vi "WSVCAP SHL Host LL Manage FPGA Top Level Controls Core.vi"(0 "Value In":variant, 1 "FPGA VI Reference (Init Only)":T2, 7 "FPGA Top Level Control":T3=enum."Read Status Flag", 11 "error in (no error)":errorcluster, 12 "Simulate FPGA (Init Only)":bool=TRUE, 13 "Operation":T4, 14 "FPGA":T1) -> (4 "Value Out":variant, 15 "error out":errorcluster)   [LabVIEW 2017]
uses:
  Type Defs/WSVCAP SHL Top Level Control Operation Enum.ctl
  Type Defs/WSVCAP SHL Top Level Control Enum.ctl
  Type Defs/WSVCAP SHL FPGA Ref.ctl
  Type Defs/WSVCAP SHL FPGA Enum.ctl
  user.lib/Utilities/Type Defs/MISC IO Choice Enum.ctl
  Type Defs/Top Level Controls Core Cluster.ctl
  Type Defs/WSVCAP SHL Gatekeeper Operation Enum.ctl
  Type Defs/WSVCAP SHL State.ctl
  Type Defs/WSVCAP SHL Transaction Enum.ctl
  <vilib>/Utility/error.llb/Error Cluster From Error Code.vi
  <vilib>/rvi/errors/niLvFpgaAdjustHostInterfaceError.vi
  <vilib>/rvi/interface/nirviReadWriteControl/nirviReadWriteControl.xnode
  FPGA Bitfiles/WSVCAPShell_WiSpryFPGA1_WSVCAPSHLFPGATLT_ffr+nD2N+rA.lvbitx
  NiFpgaLv.dll
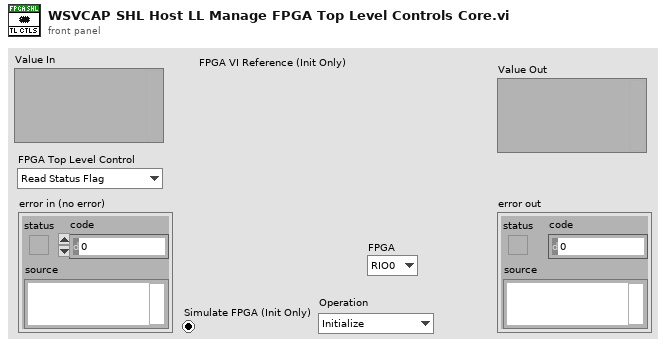
[diagram p1: front panel]
types:
  T1 = typedef "WSVCAP SHL FPGA Enum.ctl" = enum16{"RIO0", "RIO1"}
  T2 = typedef "WSVCAP SHL FPGA Ref.ctl" = refnum<k20>
  T3 = typedef "WSVCAP SHL Top Level Control Enum.ctl" = enum16{"Start", "Cmd", "Transaction", "Wait Ticks", "Socket Mask", "UUT Set", "Slave Address", "Sub Address", "Bytes to Write", "Bytes to Read", "Write Data", "Write Flag", "Read Data", "Read Flag", "Ack Read", "Read Status Flag", "Ack Read Status", "Status", "Cycle Count", "Stop Cycle", "Exit"}
  T4 = typedef "WSVCAP SHL Top Level Control Operation Enum.ctl" = enum16{"Initialize", "Set Control", "Read Control", "Close"}
  T5 = typedef "WSVCAP SHL Gatekeeper Operation Enum.ctl" = enum16{"Initialize", "Lock", "Unlock", "Close"}
  T6 = typedef "Top Level Controls Core Cluster.ctl" = cluster{"Ctl Refs":refnum<vi>[], "FPGA VI Ref":T2, "Simulate":bool}
  T7 = typedef "MISC IO Choice Enum.ctl" = enum16{"Read", "Write"}
  T8 = typedef "WSVCAP SHL State.ctl" = enum8{"Idle", "Transfer Data"}
  T9 = typedef "WSVCAP SHL Transaction Enum.ctl" = enum16{"I2C-Read Data", "I2C-Write Data", "RFFE-Ext Write", "RFFE-Ext Read"}
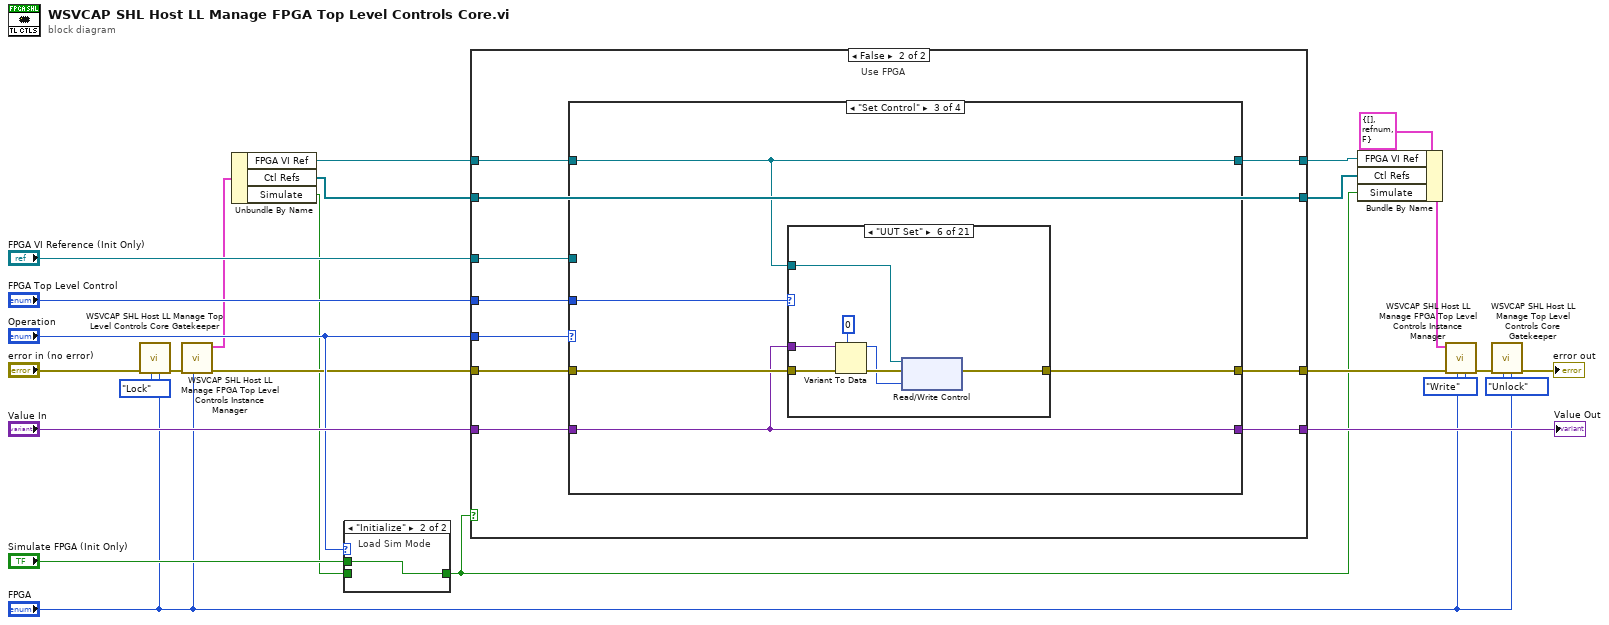
[diagram p0: block diagram]
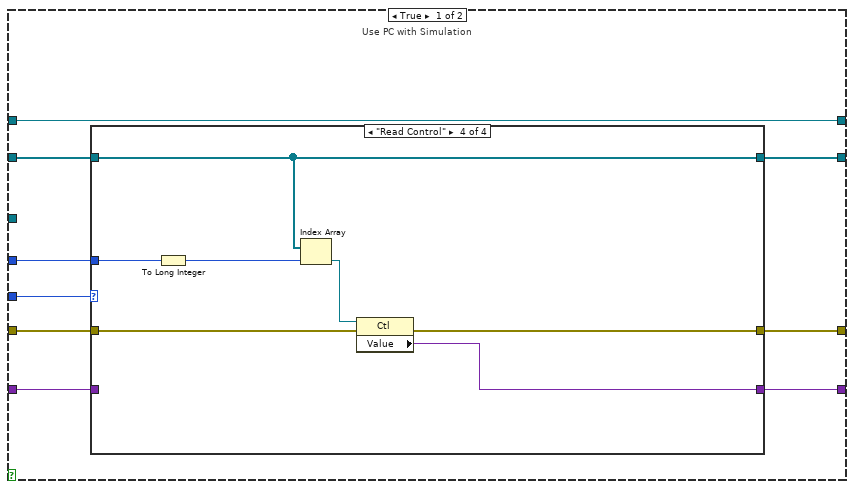
[diagram p2: hidden frame]
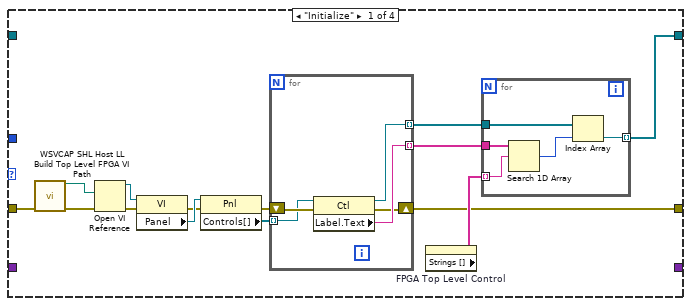
[diagram p3: hidden frame]
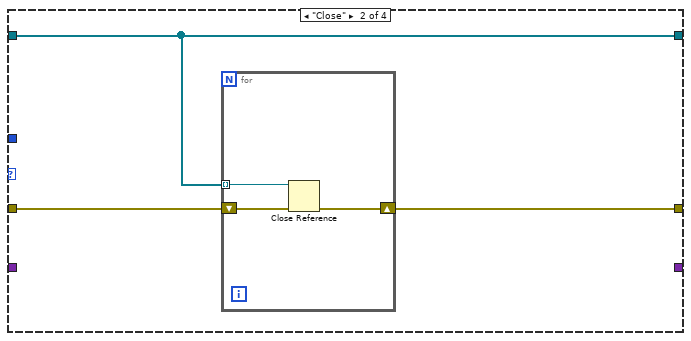
[diagram p4: hidden frame]
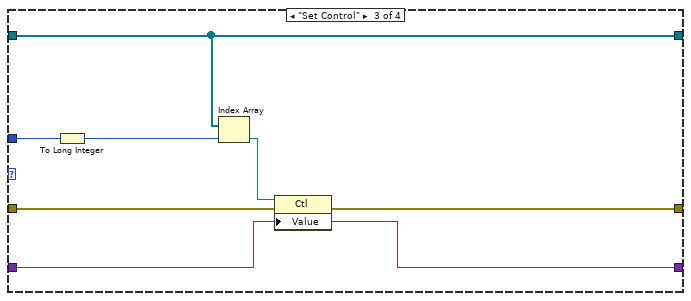
[diagram p5: hidden frame]
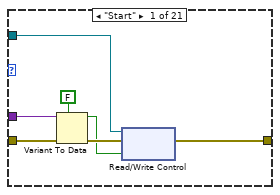
[diagram p8: hidden frame]
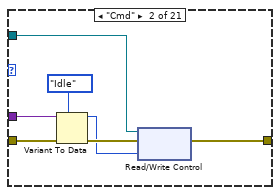
[diagram p9: hidden frame]
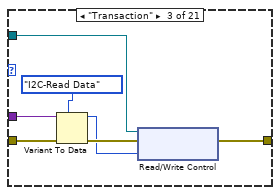
[diagram p10: hidden frame]
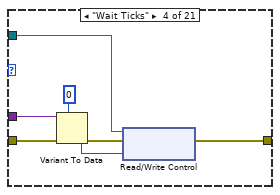
[diagram p11: hidden frame]
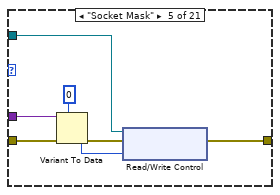
[diagram p12: hidden frame]
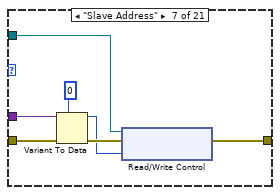
[diagram p13: hidden frame]
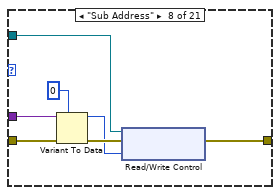
[diagram p14: hidden frame]
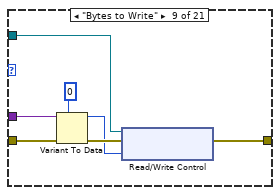
[diagram p15: hidden frame]
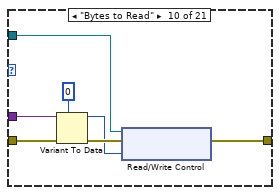
[diagram p16: hidden frame]
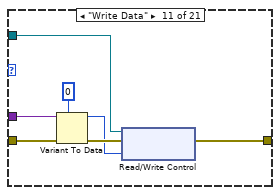
[diagram p17: hidden frame]
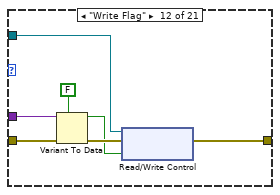
[diagram p18: hidden frame]
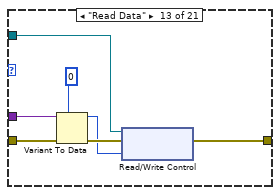
[diagram p19: hidden frame]
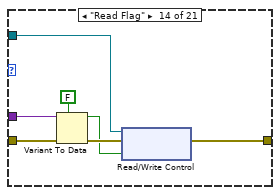
[diagram p20: hidden frame]
diagram:
  n1 = call "WSVCAP SHL Host LL Manage Top Level Controls Core Gatekeeper.vi"("FPGA"="FPGA", "Operation"=WSVCAP_SHL_Gatekeeper_Operation_Enum."Lock", "error in (no error)"="error in (no error)") -> ("error out"=w6:errorcluster)  [unwired: 8 in]
  n2 = call "WSVCAP SHL Host LL Manage FPGA Top Level Controls Instance Manager.vi"("FPGA"="FPGA", "error in (no error)"=w6) -> ("error out"=w15:errorcluster, "Top Level Controls Out"=w19:T6)  [unwired: 8 in]
  n3 = Unbundle By Name(w19) -> ("FPGA VI Ref"=w18:T2, "Ctl Refs"=w17:refnum<vi>[], "Simulate"=w9:bool)
  n4 = case shown="\"Initialize\"" "Operation" {
    tunnel: [w26 w27] -> w8
    tunnel: "Simulate FPGA (Init Only)" -> [_ w27]
    tunnel: w9 -> [w26 _]
    frame Default {
    }
    frame "Initialize" {
      # "Load Sim Mode"
    }
  }
  n5 = case shown="False" w8 {
    tunnel: "Operation" -> [w36 w90]
    tunnel: [w35 w89] -> w14
    tunnel: w15 -> [w34 w88]
    tunnel: [w33 w87] -> w25
    tunnel: "Value In" -> [w32 w86]
    tunnel: "FPGA Top Level Control" -> [w31 w85]
    tunnel: "FPGA VI Reference (Init Only)" -> [_ w84]
    tunnel: [w30 w81] -> w11
    tunnel: w17 -> [w29 w81]
    tunnel: w18 -> [w28 w83]
    tunnel: [w28 w82] -> w12
    frame True {
      # "Use PC with Simulation"
      n6 = case shown="\"Read Control\"" w36 {
        tunnel: [w44 w63 w73 w80] -> w30
        tunnel: w29 -> [_ w63 w73 w80]
        tunnel: [w40 w62 w70 w77] -> w35
        tunnel: w34 -> [w39 w61 w71 w78]
        tunnel: [_ _ w69 w76] -> w33
        tunnel: w32 -> [_ _ w69 _]
        tunnel: w31 -> [_ _ w68 w75]
        frame "Initialize" {
          n7 = call "WSVCAP SHL Host LL Build Top Level FPGA VI Path.vi"("Error In (no error)"=w39) -> ("Top Level FPGA VI Path"=w37:path, "Error Out"=w38:errorcluster)  [unwired: 13 in]
          n8 = Open VI Reference(vi path=w37, error in (no error)=w38) -> (vi reference=w50:refnum<vi>, error out=w43:errorcluster)  [unwired: 4 in]
          n9 = property class="VI"(reference=w50, error in=w43) -> (error out=w42:errorcluster, "Panel"=w49:refnum<vi>)  [unwired: 1 out]
          n10 = property class="Pnl"(reference=w49, error in=w42) -> (error out=w41:errorcluster, "Controls[]"=w48:refnum<vi>[])  [unwired: 1 out]
          n11 = for {
            tunnel: w48 -> [w56] mode=indexing
            tunnel: [w60] -> w45 mode=indexing
            tunnel: [w59] -> w47 mode=indexing
            shift-right: [w57] -> w40
            shift-left: w41 -> [w58]
            n12 = property class="Ctl"(reference=w56, error in=w58) -> (reference out=w60:refnum<vi>, error out=w57:errorcluster, "Label.Text"=w59:string)
          }
          n13 = property on="FPGA Top Level Control" class="Enum (strict)"() -> ("Strings []"=w46:string[])  [unwired: 2 in, 2 out]
          n14 = for {
            tunnel: w47 -> [w55]
            tunnel: w46 -> [w54] mode=indexing
            tunnel: w45 -> [w53]
            tunnel: [w52] -> w44 mode=indexing
            n15 = Search 1D Array(1D array=w55, element=w54) -> (index of element=w51:i32)  [unwired: 1 in]
            n16 = Index Array(array=w53, index=w51) -> (element=w52:refnum<vi>)
          }
        }
        frame "Close" {
          n17 = for {
            tunnel: w63 -> [w66] mode=indexing
            shift-right: [w65] -> w62
            shift-left: w61 -> [w64]
            n18 = Close Reference(reference=w66, error in (no error)=w64) -> (error out=w65:errorcluster)
          }
        }
        frame "Set Control" {
          n19 = To Long Integer(number=w68) -> (32bit integer=w67:i32)
          n20 = Index Array(array=w73, index=w67) -> (element=w72:refnum<vi>)
          n21 = property class="Ctl"(reference=w72, error in=w71, "Value"=w69) -> (error out=w70:errorcluster)  [unwired: 1 out]
        }
        frame "Read Control" {
          n22 = To Long Integer(number=w75) -> (32bit integer=w74:i32)
          n23 = Index Array(array=w80, index=w74) -> (element=w79:refnum<vi>)
          n24 = property class="Ctl"(reference=w79, error in=w78) -> (error out=w77:errorcluster, "Value"=w76:variant)  [unwired: 1 out]
        }
      }
    }
    frame False {
      # "Use FPGA"
      n25 = case shown="\"Set Control\"" w90 {
        tunnel: [w91 w94 w98 w249] -> w89
        tunnel: w88 -> [w91 w94 w99 w250]
        tunnel: [_ _ w96 w246] -> w87
        tunnel: w86 -> [_ _ w96 _]
        tunnel: w85 -> [_ _ w97 w248]
        tunnel: [w92 w93 w95 w247] -> w82
        tunnel: w83 -> [_ w93 w95 w247]
        tunnel: w84 -> [w92 _ _ _]
        frame "Initialize" {
        }
        frame "Close" {
        }
        frame "Set Control" {
          n26 = case shown="\"UUT Set\"" w97 {
            tunnel: w95 -> [w106 w113 w120 w127 w134 w141 w148 w155 w162 w169 w176 w183 w190 w197 w204 w211 w218 w225 w231 w238 w245]
            tunnel: w99 -> [w105 w112 w119 w126 w133 w140 w147 w154 w161 w168 w175 w182 w189 w196 w203 w210 w217 w224 w230 w237 w244]
            tunnel: [w103 w110 w117 w124 w131 w138 w145 w152 w159 w166 w173 w180 w187 w194 w201 w208 w215 w222 w228 w235 w242] -> w98
            tunnel: w96 -> [w102 w109 w116 w123 w130 w137 w144 w151 w158 w165 w172 w179 w186 w193 w200 w207 w214 w221 w227 w234 w241]
            frame "Start" {
              n27 = Variant To Data(error in=w105, type=FALSE ("SPI_CPOL"), Variant=w102) -> (data=w101:bool, error out=w104:errorcluster)
              n28 = xnode "Read/Write Control"("FPGA VI Reference In"=w106, "error in"=w104, "Start"=w101) -> ("error out"=w103:errorcluster)  [unwired: 1 out]
            }
            frame "Cmd" {
              n29 = Variant To Data(error in=w112, type=WSVCAP_SHL_State."Idle" ("SPI_Cmd"), Variant=w109) -> (data=w107:T8, error out=w111:errorcluster)
              n30 = xnode "Read/Write Control"("FPGA VI Reference In"=w113, "error in"=w111, "Cmd"=w107) -> ("error out"=w110:errorcluster)  [unwired: 1 out]
            }
            frame "Transaction" {
              n31 = Variant To Data(error in=w119, type=WSVCAP_SHL_Transaction_Enum."I2C-Read Data" ("Transaction"), Variant=w116) -> (data=w114:T9, error out=w118:errorcluster)
              n32 = xnode "Read/Write Control"("FPGA VI Reference In"=w120, "error in"=w118, "Transaction"=w114) -> ("error out"=w117:errorcluster)  [unwired: 1 out]
            }
            frame "Wait Ticks" {
              n33 = Variant To Data(error in=w126, type=u32 0 ("I2C_Clock Divider"), Variant=w123) -> (data=w122:u32, error out=w125:errorcluster)
              n34 = xnode "Read/Write Control"("FPGA VI Reference In"=w127, "error in"=w125, "Wait Ticks"=w122) -> ("error out"=w124:errorcluster)  [unwired: 1 out]
            }
            frame "Socket Mask" {
              n35 = Variant To Data(error in=w133, type=u64 0 ("I2C_Clock Divider"), Variant=w130) -> (data=w129:u64, error out=w132:errorcluster)
              n36 = xnode "Read/Write Control"("FPGA VI Reference In"=w134, "error in"=w132, "Socket Mask"=w129) -> ("error out"=w131:errorcluster)  [unwired: 1 out]
            }
            frame "UUT Set" {
              n37 = Variant To Data(error in=w140, type=u8 0 ("I2C_Clock Divider"), Variant=w137) -> (data=w135:u8, error out=w139:errorcluster)
              n38 = xnode "Read/Write Control"("FPGA VI Reference In"=w141, "error in"=w139, "UUT Set"=w135) -> ("error out"=w138:errorcluster)  [unwired: 1 out]
            }
            frame "Slave Address" {
              n39 = Variant To Data(error in=w147, type=u8 0 ("I2C_Slave Address"), Variant=w144) -> (data=w143:u8, error out=w146:errorcluster)
              n40 = xnode "Read/Write Control"("FPGA VI Reference In"=w148, "error in"=w146, "Slave Address"=w143) -> ("error out"=w145:errorcluster)  [unwired: 1 out]
            }
            frame "Sub Address" {
              n41 = Variant To Data(error in=w154, type=u8 0 ("SPI_CS"), Variant=w151) -> (data=w149:u8, error out=w153:errorcluster)
              n42 = xnode "Read/Write Control"("FPGA VI Reference In"=w155, "error in"=w153, "Sub Address"=w149) -> ("error out"=w152:errorcluster)  [unwired: 1 out]
            }
            frame "Bytes to Write" {
              n43 = Variant To Data(error in=w161, type=u8 0 ("SPI_Clock Divider"), Variant=w158) -> (data=w157:u8, error out=w160:errorcluster)
              n44 = xnode "Read/Write Control"("FPGA VI Reference In"=w162, "error in"=w160, "Bytes to Write"=w157) -> ("error out"=w159:errorcluster)  [unwired: 1 out]
            }
            frame "Bytes to Read" {
              n45 = Variant To Data(error in=w168, type=u8 0 ("SPI_Total Bytes"), Variant=w165) -> (data=w164:u8, error out=w167:errorcluster)
              n46 = xnode "Read/Write Control"("FPGA VI Reference In"=w169, "error in"=w167, "Bytes to Read"=w164) -> ("error out"=w166:errorcluster)  [unwired: 1 out]
            }
            frame "Write Data" {
              n47 = Variant To Data(error in=w175, type=u64 0 ("SPI_Total Bytes"), Variant=w172) -> (data=w171:u64, error out=w174:errorcluster)
              n48 = xnode "Read/Write Control"("FPGA VI Reference In"=w176, "error in"=w174, "Write Data"=w171) -> ("error out"=w173:errorcluster)  [unwired: 1 out]
            }
            frame "Write Flag" {
              n49 = Variant To Data(error in=w182, type=FALSE, Variant=w179) -> (data=w178:bool, error out=w181:errorcluster)
              n50 = xnode "Read/Write Control"("FPGA VI Reference In"=w183, "error in"=w181, "Write Flag"=w178) -> ("error out"=w180:errorcluster)  [unwired: 1 out]
            }
            frame "Read Data" {
              n51 = Variant To Data(error in=w189, type=u64 0 ("I2C_Read Data"), Variant=w186) -> (data=w184:u64, error out=w188:errorcluster)
              n52 = xnode "Read/Write Control"("FPGA VI Reference In"=w190, "error in"=w188, "Read Data"=w184) -> ("error out"=w187:errorcluster)  [unwired: 1 out]
            }
            frame "Read Flag" {
              n53 = Variant To Data(error in=w196, type=FALSE ("SPI_CPOL"), Variant=w193) -> (data=w191:bool, error out=w195:errorcluster)
              n54 = xnode "Read/Write Control"("FPGA VI Reference In"=w197, "error in"=w195, "Read Flag"=w191) -> ("error out"=w194:errorcluster)  [unwired: 1 out]
            }
            frame "Ack Read" {
              n55 = Variant To Data(error in=w203, type=FALSE ("SPI_CPOL"), Variant=w200) -> (data=w199:bool, error out=w202:errorcluster)
              n56 = xnode "Read/Write Control"("FPGA VI Reference In"=w204, "error in"=w202, "Ack Read"=w199) -> ("error out"=w201:errorcluster)  [unwired: 1 out]
            }
            frame "Read Status Flag" {
              n57 = Variant To Data(error in=w210, type=FALSE ("SPI_CPOL"), Variant=w207) -> (data=w206:bool, error out=w209:errorcluster)
              n58 = xnode "Read/Write Control"("FPGA VI Reference In"=w211, "error in"=w209, "Read Status Flag"=w206) -> ("error out"=w208:errorcluster)  [unwired: 1 out]
            }
            frame "Ack Read Status" {
              n59 = Variant To Data(error in=w217, type=FALSE ("SPI_CPOL"), Variant=w214) -> (data=w213:bool, error out=w216:errorcluster)
              n60 = xnode "Read/Write Control"("FPGA VI Reference In"=w218, "error in"=w216, "Ack Read Status"=w213) -> ("error out"=w215:errorcluster)  [unwired: 1 out]
            }
            frame "Status" {
              n61 = Variant To Data(error in=w224, type=0 ("I2C_Status"), Variant=w221) -> (data=w219:i32, error out=w223:errorcluster)
              n62 = xnode "Read/Write Control"("FPGA VI Reference In"=w225, "error in"=w223, "Status"=w219) -> ("error out"=w222:errorcluster)  [unwired: 1 out]
            }
            frame "Cycle Count" {
              w226 = u64 0 ("Cycle Count")
              n63 = Variant To Data(error in=w230, type=w226, Variant=w227) -> (error out=w229:errorcluster)  [unwired: 1 out]
              n64 = xnode "Read/Write Control"("FPGA VI Reference In"=w231, "error in"=w229, "Cycle Count"=w226) -> ("error out"=w228:errorcluster)  [unwired: 1 out]
            }
            frame "Stop Cycle" {
              n65 = Variant To Data(error in=w237, type=FALSE ("SPI_CPOL"), Variant=w234) -> (data=w233:bool, error out=w236:errorcluster)
              n66 = xnode "Read/Write Control"("FPGA VI Reference In"=w238, "error in"=w236, "Stop Cycle"=w233) -> ("error out"=w235:errorcluster)  [unwired: 1 out]
            }
            frame "Exit" {
              n67 = Variant To Data(error in=w244, type=FALSE ("I2C_Exit"), Variant=w241) -> (data=w240:bool, error out=w243:errorcluster)
              n68 = xnode "Read/Write Control"("FPGA VI Reference In"=w245, "error in"=w243, "Exit"=w240) -> ("error out"=w242:errorcluster)  [unwired: 1 out]
            }
          }
        }
        frame "Read Control" {
          n69 = case shown="\"UUT Set\"" w248 {
            tunnel: w247 -> [w255 w260 w265 w270 w275 w280 w285 w290 w295 w300 w305 w310 w315 w320 w325 w330 w335 w340 w345 w350 w355]
            tunnel: w250 -> [w253 w258 w263 w266 w271 w276 w281 w286 w293 w298 w302 w308 w313 w318 w323 w328 w333 w338 w343 w348 w353]
            tunnel: [w254 w259 w264 w269 w274 w279 w284 w289 w294 w299 w304 w309 w314 w319 w324 w329 w334 w339 w344 w349 w354] -> w249
            tunnel: [w251 w256 w262 w267 w272 w277 w282 w287 w291 w296 w301 w306 w311 w316 w321 w326 w331 w336 w341 w346 w351] -> w246
            frame "Start" {
              n70 = xnode "Read/Write Control"("FPGA VI Reference In"=w255, "error in"=w253) -> ("error out"=w254:errorcluster, "Start"=w252:bool)  [unwired: 1 out]
              n71 = To Variant(anything=w252) -> (Variant=w251:variant)
            }
            frame "Cmd" {
              n72 = xnode "Read/Write Control"("FPGA VI Reference In"=w260, "error in"=w258) -> ("error out"=w259:errorcluster, "Cmd"=w257:T8)  [unwired: 1 out]
              n73 = To Variant(anything=w257) -> (Variant=w256:variant)
            }
            frame "Transaction" {
              n74 = xnode "Read/Write Control"("FPGA VI Reference In"=w265, "error in"=w263) -> ("error out"=w264:errorcluster, "Transaction"=w261:T9)  [unwired: 1 out]
              n75 = To Variant(anything=w261) -> (Variant=w262:variant)
            }
            frame "Wait Ticks" {
              n76 = xnode "Read/Write Control"("FPGA VI Reference In"=w270, "error in"=w266) -> ("error out"=w269:errorcluster, "Wait Ticks"=w268:u32)  [unwired: 1 out]
              n77 = To Variant(anything=w268) -> (Variant=w267:variant)
            }
            frame "Socket Mask" {
              n78 = xnode "Read/Write Control"("FPGA VI Reference In"=w275, "error in"=w271) -> ("error out"=w274:errorcluster, "Socket Mask"=w273:u64)  [unwired: 1 out]
              n79 = To Variant(anything=w273) -> (Variant=w272:variant)
            }
            frame "UUT Set" {
              n80 = xnode "Read/Write Control"("FPGA VI Reference In"=w280, "error in"=w276) -> ("error out"=w279:errorcluster, "UUT Set"=w278:u8)  [unwired: 1 out]
              n81 = To Variant(anything=w278) -> (Variant=w277:variant)
            }
            frame "Cycle Count" {
              n82 = xnode "Read/Write Control"("FPGA VI Reference In"=w285, "error in"=w281) -> ("error out"=w284:errorcluster, "Cycle Count"=w283:u64)  [unwired: 1 out]
              n83 = To Variant(anything=w283) -> (Variant=w282:variant)
            }
            frame "Stop Cycle" {
              n84 = xnode "Read/Write Control"("FPGA VI Reference In"=w290, "error in"=w286) -> ("error out"=w289:errorcluster, "Stop Cycle"=w288:bool)  [unwired: 1 out]
              n85 = To Variant(anything=w288) -> (Variant=w287:variant)
            }
            frame "Slave Address" {
              n86 = xnode "Read/Write Control"("FPGA VI Reference In"=w295, "error in"=w293) -> ("error out"=w294:errorcluster, "Slave Address"=w292:u8)  [unwired: 1 out]
              n87 = To Variant(anything=w292) -> (Variant=w291:variant)
            }
            frame "Sub Address" {
              n88 = xnode "Read/Write Control"("FPGA VI Reference In"=w300, "error in"=w298) -> ("error out"=w299:errorcluster, "Sub Address"=w297:u8)  [unwired: 1 out]
              n89 = To Variant(anything=w297) -> (Variant=w296:variant)
            }
            frame "Bytes to Write" {
              n90 = xnode "Read/Write Control"("FPGA VI Reference In"=w305, "error in"=w302) -> ("error out"=w304:errorcluster, "Bytes to Write"=w303:u8)  [unwired: 1 out]
              n91 = To Variant(anything=w303) -> (Variant=w301:variant)
            }
            frame "Bytes to Read" {
              n92 = xnode "Read/Write Control"("FPGA VI Reference In"=w310, "error in"=w308) -> ("error out"=w309:errorcluster, "Bytes to Read"=w307:u8)  [unwired: 1 out]
              n93 = To Variant(anything=w307) -> (Variant=w306:variant)
            }
            frame "Write Data" {
              n94 = xnode "Read/Write Control"("FPGA VI Reference In"=w315, "error in"=w313) -> ("error out"=w314:errorcluster, "Write Data"=w312:u64)  [unwired: 1 out]
              n95 = To Variant(anything=w312) -> (Variant=w311:variant)
            }
            frame "Write Flag" {
              n96 = xnode "Read/Write Control"("FPGA VI Reference In"=w320, "error in"=w318) -> ("error out"=w319:errorcluster, "Write Flag"=w317:bool)  [unwired: 1 out]
              n97 = To Variant(anything=w317) -> (Variant=w316:variant)
            }
            frame "Read Data" {
              n98 = xnode "Read/Write Control"("FPGA VI Reference In"=w325, "error in"=w323) -> ("error out"=w324:errorcluster, "Read Data"=w322:u64)  [unwired: 1 out]
              n99 = To Variant(anything=w322) -> (Variant=w321:variant)
            }
            frame "Read Flag" {
              n100 = xnode "Read/Write Control"("FPGA VI Reference In"=w330, "error in"=w328) -> ("error out"=w329:errorcluster, "Read Flag"=w327:bool)  [unwired: 1 out]
              n101 = To Variant(anything=w327) -> (Variant=w326:variant)
            }
            frame "Ack Read" {
              n102 = xnode "Read/Write Control"("FPGA VI Reference In"=w335, "error in"=w333) -> ("error out"=w334:errorcluster, "Ack Read"=w332:bool)  [unwired: 1 out]
              n103 = To Variant(anything=w332) -> (Variant=w331:variant)
            }
            frame "Read Status Flag" {
              n104 = xnode "Read/Write Control"("FPGA VI Reference In"=w340, "error in"=w338) -> ("error out"=w339:errorcluster, "Read Status Flag"=w337:bool)  [unwired: 1 out]
              n105 = To Variant(anything=w337) -> (Variant=w336:variant)
            }
            frame "Ack Read Status" {
              n106 = xnode "Read/Write Control"("FPGA VI Reference In"=w345, "error in"=w343) -> ("error out"=w344:errorcluster, "Ack Read Status"=w342:bool)  [unwired: 1 out]
              n107 = To Variant(anything=w342) -> (Variant=w341:variant)
            }
            frame "Status" {
              n108 = xnode "Read/Write Control"("FPGA VI Reference In"=w350, "error in"=w348) -> ("error out"=w349:errorcluster, "Status"=w347:i32)  [unwired: 1 out]
              n109 = To Variant(anything=w347) -> (Variant=w346:variant)
            }
            frame "Exit" {
              n110 = xnode "Read/Write Control"("FPGA VI Reference In"=w355, "error in"=w353) -> ("error out"=w354:errorcluster, "Exit"=w352:bool)  [unwired: 1 out]
              n111 = To Variant(anything=w352) -> (Variant=w351:variant)
            }
          }
        }
      }
    }
  }
  "Value Out" <- w25
  n112 = Bundle By Name(cluster=T6 {"Ctl Refs"=[], "FPGA VI Ref"=refnum, "Simulate"=FALSE} ("Top Level Controls Out"), "FPGA VI Ref"=w12, "Ctl Refs"=w11, "Simulate"=w8) -> (w10:T6)
  n113 = call "WSVCAP SHL Host LL Manage FPGA Top Level Controls Instance Manager.vi"("I/O Choice (read)"=MISC_IO_Choice_Enum."Write", "FPGA"="FPGA", "error in (no error)"=w14, "Top Level Controls In"=w10) -> ("error out"=w5:errorcluster)  [unwired: 6 in, 1 out]
  n114 = call "WSVCAP SHL Host LL Manage Top Level Controls Core Gatekeeper.vi"("FPGA"="FPGA", "Operation"=WSVCAP_SHL_Gatekeeper_Operation_Enum."Unlock", "error in (no error)"=w5) -> ("error out"=→"error out":errorcluster)  [unwired: 8 in]
